vi "Compare Previous INSERT.vi"(8 "error in":errorcluster, 11 "Data":variant) -> (0 "error out":errorcluster, 1 "Some Different":bool, 2 "All Different":bool, 3 "Data out":variant)   [LabVIEW 2019, in "LV-Data.PGSQL.lvclass"]
uses:
  LV-Data.PGSQL.lvclass
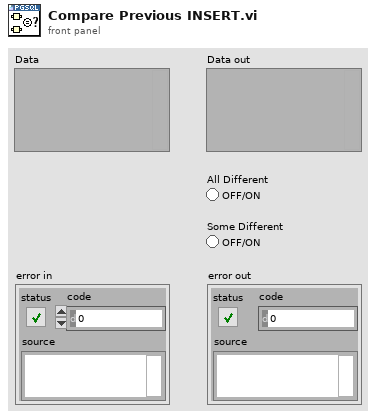
[diagram p1: front panel]
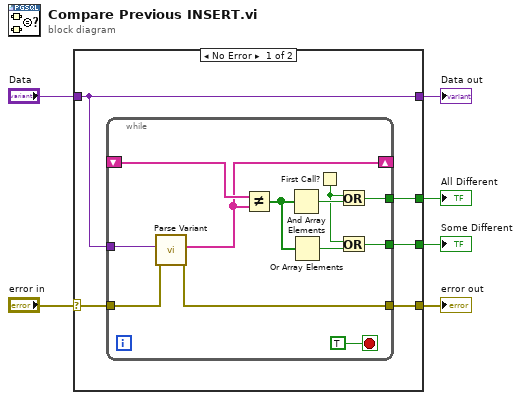
[diagram p0: block diagram]
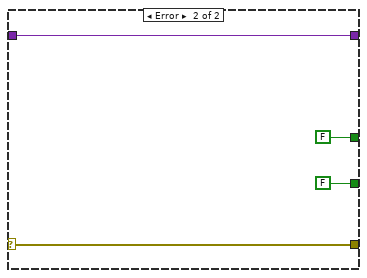
[diagram p2: hidden frame]
diagram:
  n1 = case shown="No Error" "error in" {
    selector: "error in" -> [w7 w26]
    tunnel: [w11 w26] -> w6
    tunnel: [w10 FALSE] -> w5
    tunnel: [w9 FALSE] -> w4
    tunnel: "Data" -> [w8 w27]
    tunnel: [w8 w27] -> w1
    frame No Error {
      n2 = while {
        shift-right: [w12] -> _
        shift-left: _ -> [w13]
        tunnel: w8 -> [w23]
        tunnel: w7 -> [w14]
        tunnel: [w15] -> w11
        tunnel: [w18] -> w10
        tunnel: [w17] -> w9
        stop <- TRUE stop-if-true
        n3 = call "Parse Variant.vi"("error in"=w14, "Data"=w23) -> ("error out"=w15:errorcluster, "Data"=w12:string[])  [unwired: 5 in, 3 out]
        n4 = Not Equal?(x=w13, y=w12) -> (x != y?=w21:bool[])
        n5 = And Array Elements(Boolean array=w21) -> (logical AND=w19:bool)
        n6 = Or Array Elements(Boolean array=w21) -> (logical OR=w20:bool)
        n7 = First Call?() -> (First Call?: T/F=w16:bool)
        n8 = Or(x=w16, y=w19) -> (x .or. y?=w17:bool)
        n9 = Or(x=w16, y=w20) -> (x .or. y?=w18:bool)
      }
    }
    frame Error {
    }
  }
  "error out" <- w6
  "All Different" <- w4
  "Some Different" <- w5
  "Data out" <- w1
